vi "VirtualBench_I2C Bus Mastering.vi"() -> ()   [LabVIEW 2015]
doc: "This example demonstrates how to write to an I2C bus and then read back from an I2C Slave.\n\nYou can use VirtualBench to master an I2C bus. When you configure an I2C bus, a set of lines are reserved for the bus and each line's direction is automatically configured. By default, digital lines used in I2C buses have no pull resistors connected. A 10 kohm pull-up resistor to 3.3V can be programmatically connected to the lines on the bus.\n\ndig/6: SCL (Serial Clock) output\ndig/7: SDA (Serial Data) input/output"
uses:
  <vilib>/RAFA Solutions/Rainbow Flat UI Controls Kit (Light)/Boolean/Round Led.ctl
  <vilib>/Utility/error.llb/DialogType.ctl
  <vilib>/VirtualBench/_I2C Configure Bus0.vi
  <vilib>/VirtualBench/VirtualBench.lvlib
  <vilib>/RAFA Solutions/Rainbow Flat UI Controls Kit (Light)/Rainbow Light.lvlib
panel:
  out "LED Status":T1
  in  "Cancel Button":bool
  in  "Threshold (F)":dbl(slide) scale=50.0..100.0
  out "Thermometer (F)":dbl(slide)=72.6517080078125 scale=0.0..100.0
  out "Combined Boolean Array":bool[](array[boolean])=[FALSE, FALSE, FALSE, TRUE, FALSE, TRUE, FALSE, FALSE, TRUE, FALSE, TRUE, FALSE, FALSE, TRUE, TRUE, FALSE]
  in  "Lines":tag="dig/0:1"
  in  "Digital IO Channel":tag="VB8012-3060439/dig/0:1" caption="Bus"
  in  "Enable Pull Ups":bool caption="Enable Pull Ups (no change)"
  in  "Address":u16=64 format="%x"
  in  "Write Data":u8[](array[numeric])=[227] format="%x"
  out "Results":u8[](array[numeric])=[101, 168, 103, 255, 255, 255, 255, 255] caption="Read Data" format="%x"
  in  "Number of Bytes To Read":i32=3 caption="Number Of Bytes To Read"
  in  "Bus Channel":tag="VB8012-3060439/i2c/0" caption="Bus"
  in  "Address Size":i32(ring) caption="Address Size (no change)" items=["7 Bits", "10 Bits"]
  in  "Clock Rate":i32(ring)=1 items=["100 kHz", "400 kHz", "1 MHz"]
  # "I2C Configuration"
  # "Data to Write"
  # "Results"
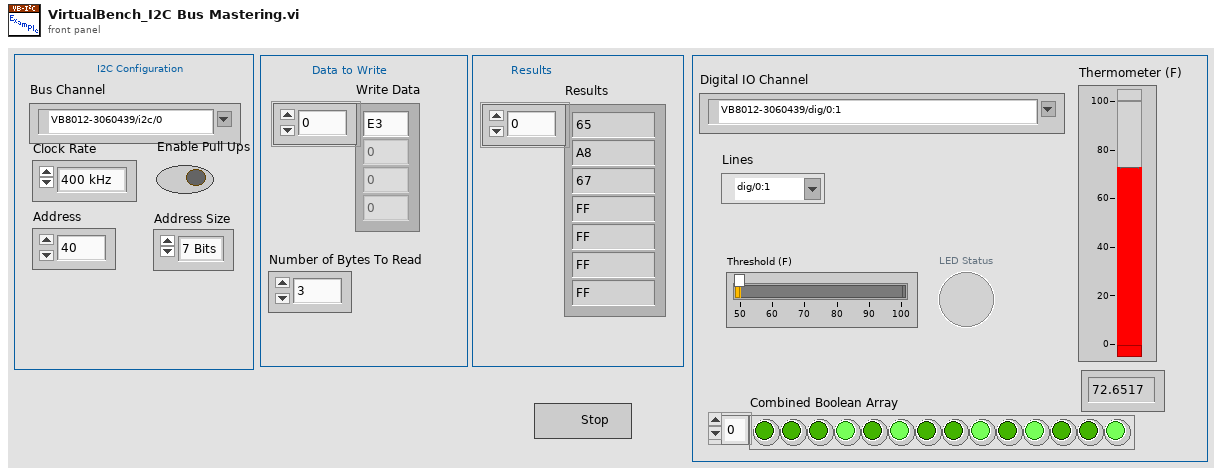
[diagram p1: front panel]
types:
  T1 = typedef "Rainbow Light.lvlib/Round Led.ctl" = bool
  T2 = typedef "DialogType.ctl" = u16
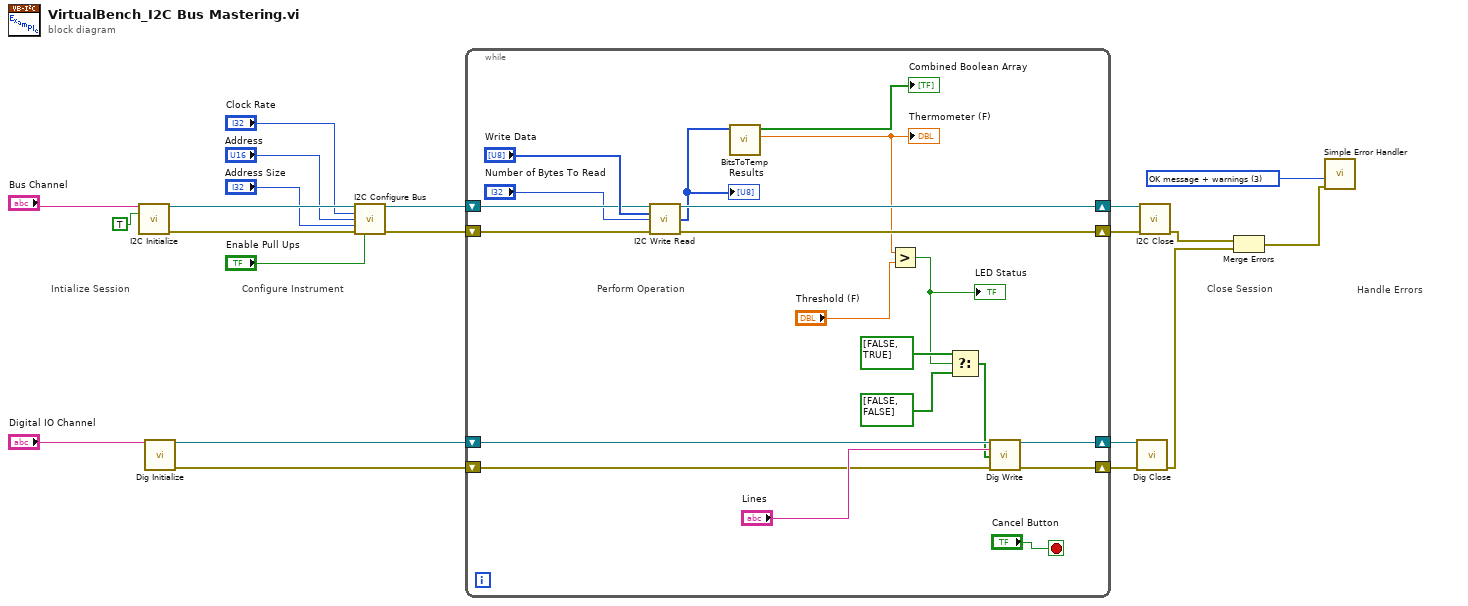
[diagram p0: block diagram]
diagram:
  w21 = T2 3 items=["no dialog", "OK message", "continue or stop message", "OK message + warnings", "continue/stop + warnings"] ("type of dialog (OK msg:1)")
  # "Handle Errors"
  # "Configure Instrument"
  # "Intialize Session"
  # "Close Session"
  n1 = call <vilib>:"I2C Initialize.vi"("Bus"="Bus Channel", "Reset"=TRUE) -> ("Instrument Handle Out"=w20:refnum<k21>, "Error Out"=w19:errorcluster)  [unwired: 12 in]
  n2 = call <vilib>:"Dig Initialize.vi"("Lines"="Digital IO Channel") -> ("Instrument Handle Out"=w7:refnum<k21>, "Error Out"=w4:errorcluster)  [unwired: 13 in]
  n3 = call-poly <vilib>:"I2C Configure Bus.vi"("Instrument Handle In"=w20, "Clock Rate"="Clock Rate", "Address"="Address", "Address Size"="Address Size", "Error In"=w19, "Enable Pull Ups"="Enable Pull Ups") -> ("Instrument Handle Out"=w13:refnum<k21>, "Error Out"=w12:errorcluster)  [unwired: 8 in]
  n4 = while {
    shift-right: [w37] -> w11
    shift-left: w13 -> [w40]
    shift-right: [w36] -> w10
    shift-left: w12 -> [w39]
    shift-right: [w32] -> w6
    shift-left: w7 -> [w34]
    shift-right: [w31] -> w5
    shift-left: w4 -> [w30]
    stop <- "Cancel Button" stop-if-true
    # "Perform Operation"
    n5 = call <vilib>:"I2C Write Read.vi"("Instrument Handle In"=w40, "Write Data"="Write Data", "Number Of Bytes To Read"="Number of Bytes To Read", "Error In"=w39) -> ("Instrument Handle Out"=w37:refnum<k21>, "Read Data"=w35:u8[], "Error Out"=w36:errorcluster)  [unwired: 8 in, 1 out]
    "Results" <- w35
    n6 = call "BitsToTemp.vi"("Raw I2C Packets"=w35) -> ("Temperature (F)"=w29:dbl, "Array"=→"Combined Boolean Array":bool[])  [unwired: 8 in, 1 out]
    "Thermometer (F)" <- w29
    n7 = Greater?(x=w29, y="Threshold (F)") -> (0:w22:bool)
    "LED Status" <- w22
    n8 = Select(t=bool[] [FALSE, TRUE] ("Data"), s=w22, f=bool[] [FALSE, FALSE] ("Data")) -> (s? t:f=w23:bool[])
    n9 = call <vilib>:"Dig Write.vi"("Instrument Handle In"=w34, "Lines"="Lines", "Data"=w23, "Error In"=w30) -> ("Instrument Handle Out"=w32:refnum<k21>, "Error Out"=w31:errorcluster)  [unwired: 10 in]
  }
  n10 = call <vilib>:"Dig Close.vi"("Instrument Handle In"=w6, "Error In"=w5) -> ("Error Out"=w1:errorcluster)  [unwired: 13 in]
  n11 = call <vilib>:"I2C Close.vi"("Instrument Handle In"=w11, "Error In"=w10) -> ("Error Out"=w3:errorcluster)  [unwired: 13 in]
  n12 = Merge Errors(w3, w1) -> (w2:errorcluster)
  n13 = call <vilib>:"Simple Error Handler.vi"("type of dialog (OK msg:1)"=w21, "error in (no error)"=w2) -> ()  [unwired: 3 in, 5 out]
